vi "07.4 Loop Shift registers with API.vi"() -> ()   [LabVIEW 2019]
uses:
  <vilib>/DAQmx/read.llb/DAQmx Read (Analog DBL 1Chan 1Samp).vi
  <vilib>/DAQmx/miscellaneous.llb/DAQmx Fill In Error Info.vi
panel:
  out "Max temperature registered":dbl format="%0.2f"
  out "Measured temperature":dbl format="%0.2f"
  out "Temperature Exceeded?":bool
  in  "Threshold temperature":dbl(slide) scale=30.0..80.0
  in  "Stop":bool
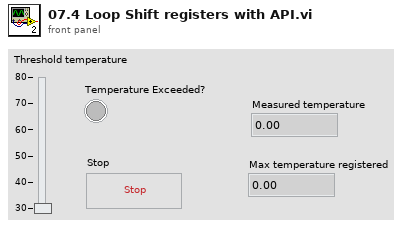
[diagram p1: front panel]
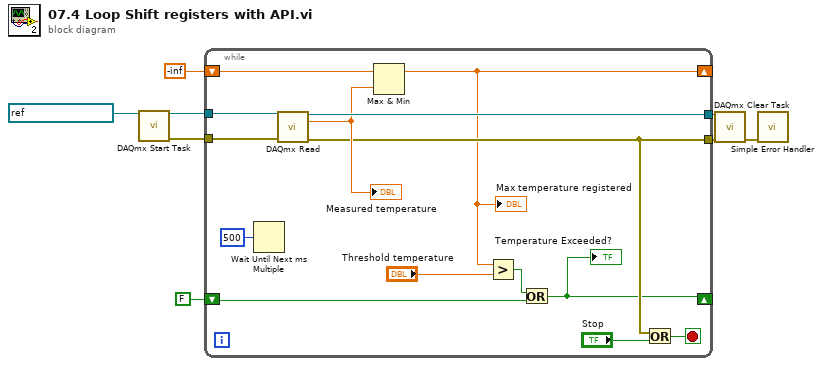
[diagram p0: block diagram]
diagram:
  n1 = call <vilib>:"DAQmx Start Task.vi"("task/channels in"=refnum<k21> "Thermocouple" ("task in")) -> ("task out"=w8:refnum<k21>, "error out"=w7:errorcluster)  [unwired: 13 in]
  n2 = while {
    tunnel: w8 -> [w21]
    tunnel: w7 -> [w22]
    tunnel: [w15] -> w6
    tunnel: [w19] -> w5
    shift-right: [w10] -> _
    shift-left: -inf -> [w18]
    shift-right: [w12] -> _
    shift-left: FALSE -> [w13]
    stop <- w20 stop-if-true
    n3 = Wait Until Next ms Multiple(millisecond multiple=u32 500) -> ()  [unwired: 1 out]
    n4 = call-poly <vilib>:"DAQmx Read.vi"("task/channels in"=w21, "error in"=w22) -> ("task out"=w19:refnum<k21>, "data"=w17:dbl, "error out"=w15:errorcluster)  [unwired: 11 in]
    "Measured temperature" <- w17
    n5 = Max & Min(x=w18, y=w17) -> (max(x,y)=w10:dbl)  [unwired: 1 out]
    "Max temperature registered" <- w10
    n6 = Greater?(x=w10, y="Threshold temperature") -> (0:w14:bool)
    n7 = Or(x=w14, y=w13) -> (x .or. y?=w12:bool)
    "Temperature Exceeded?" <- w12
    n8 = Or(x=w15, y="Stop") -> (x .or. y?=w20:bool)
  }
  n9 = call <vilib>:"DAQmx Clear Task.vi"("task in"=w5, "error in"=w6) -> ("error out"=w4:errorcluster)  [unwired: 13 in]
  n10 = call <vilib>:"Simple Error Handler.vi"("error in (no error)"=w4) -> ()  [unwired: 4 in, 5 out]
